vi "LowPassFilter.vi"(7 "Low-pass filter":T2={"Clip off ramp-up, 1/Fc"=1.0, "Double-pass in reverse"=TRUE, "IIR filter specifications"={"Topology"=enum."Butterworth", "Type"=enum."Lowpass", "Order"=1, "Lower Fc"=10000.0, "Upper Fc"=200.0, "PB Ripple"=1.0, "SB Attenuation"=60.0}} {"IIR filter specifications"."PB Ripple" format="%0.2f"; "IIR filter specifications"."Lower Fc" format="%0.2p"; "IIR filter specifications"."SB Attenuation" format="%0.2f"; "IIR filter specifications"."Upper Fc" format="%0.2p"}, 8 "error in (no error)":errorcluster, 9 "Settings":string, 11 "signal(s) in":waveform(dbl)[](array[waveform])) -> (0 "error out":errorcluster, 1 "Settings out":string, 3 "signal(s) out":waveform(dbl)[](array[waveform]), 4 "filter information":T1 {"phase H(w)"."df" format="%.2p"; "phase H(w)"."f0" format="%.2p"; "phase H(w)"."Phase H(w)" format="%.2p"; "magnitude H(w)"."df" format="%.2p"; "magnitude H(w)"."f0" format="%.2p"; "magnitude H(w)"."Mag H(w)" format="%.2p"})   [LabVIEW 2015]
uses:
  IIR Filter parameters.ctl
  <vilib>/measure/macond.llb/IIR Filter for N Chan.vi
  <vilib>/Waveform/WDTOps.llb/WDT Waveform Duration DBL.vi
  <vilib>/Waveform/WDTOps.llb/WDT Get Waveform Subset DBL.vi
  <vilib>/measure/NI_MAPro.lvlib
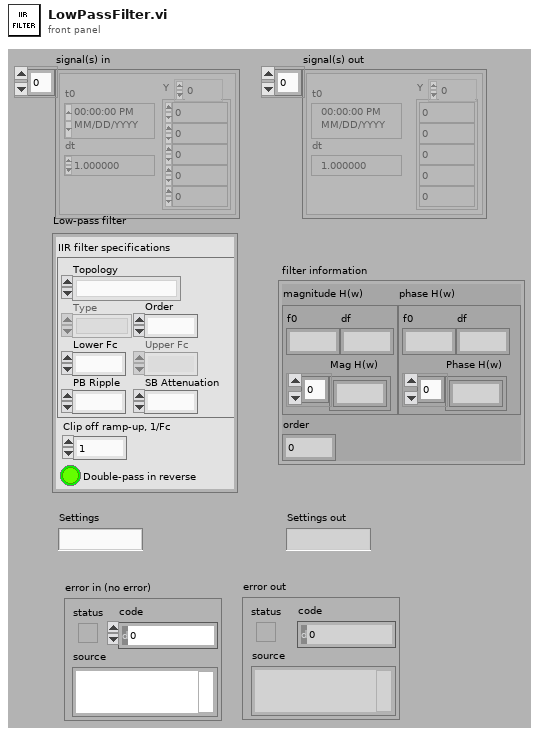
[diagram p1: front panel]
types:
  T1 = cluster{"magnitude H(w)":cluster{"f0":dbl, "df":dbl, "Mag H(w)":dbl[]}, "phase H(w)":cluster{"f0":dbl, "df":dbl, "Phase H(w)":dbl[]}, "order":i32}
  T2 = typedef "IIR Filter parameters.ctl" = cluster{"Clip off ramp-up, 1/Fc":dbl, "Double-pass in reverse":bool, "IIR filter specifications":cluster{"Topology":enum16{"Off", "Butterworth", "Chebyshev", "Inverse Chebyshev", "Elliptic", "Bessel"}, "Type":enum16{"Lowpass", "Highpass", "Bandpass", "Bandstop"}, "Order":i32, "Lower Fc":dbl, "Upper Fc":dbl, "PB Ripple":dbl, "SB Attenuation":dbl}}
  T3 = cluster{"Topology":enum16{"Off", "Butterworth", "Chebyshev", "Inverse Chebyshev", "Elliptic", "Bessel"}, "Type":enum16{"Lowpass", "Highpass", "Bandpass", "Bandstop"}, "Order":i32, "Lower Fc":dbl, "Upper Fc":dbl, "PB Ripple":dbl, "SB Attenuation":dbl}
  T4 = enum16{"Off", "Butterworth", "Chebyshev", "Inverse Chebyshev", "Elliptic", "Bessel"}
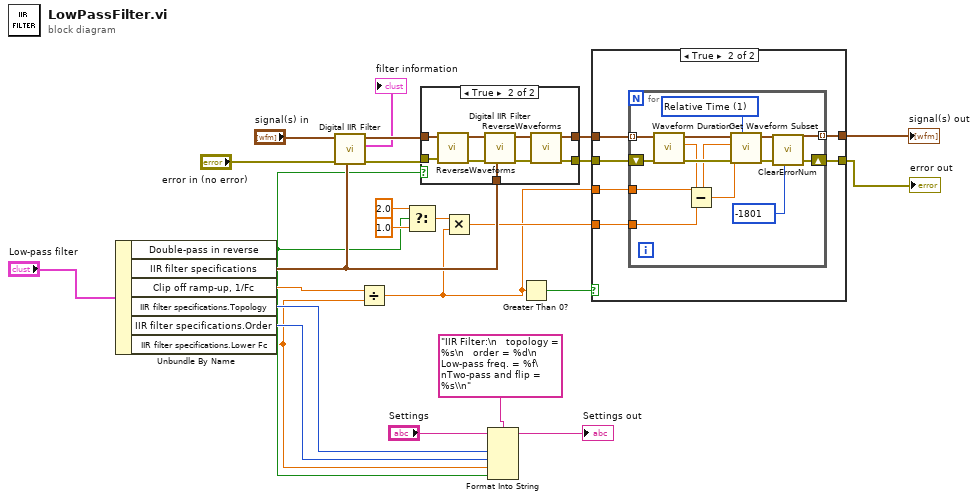
[diagram p0: block diagram]
diagram:
  n1 = Unbundle By Name("Low-pass filter") -> ("Double-pass in reverse"=w4:bool, "IIR filter specifications"=w21:T3, "Clip off ramp-up, 1/Fc"=w10:dbl, "IIR filter specifications.Topology"=w7:T4, "IIR filter specifications.Order"=w5:i32, "IIR filter specifications.Lower Fc"=w2:dbl)
  n2 = call-poly <vilib>:"Digital IIR Filter.vi"("IIR filter specifications"=w21, "error in (no error)"="error in (no error)", "signal(s) in"="signal(s) in") -> ("error out"=w24:errorcluster, "filter information"=→"filter information":T1, "signal(s) out"=w25:waveform(dbl)[])  [unwired: 3 in, 3 out]
  n3 = Divide(x=w10, y=w2) -> (x/y=w3:dbl)
  n4 = Select(t=2.0, s=w4, f=1.0) -> (s? t:f=w15:dbl)
  n5 = case shown="True" w4 {
    tunnel: w25 -> [w26 w34]
    tunnel: w24 -> [w27 w33]
    tunnel: [w27 w32] -> w19
    tunnel: [w26 w28] -> w20
    tunnel: w21 -> [_ w30]
    frame False {
    }
    frame True {
      n6 = call "ReverseWaveforms.vi"("signals in"=w34) -> ("signals out"=w29:waveform(dbl)[])  [unwired: 10 out]
      n7 = call-poly <vilib>:"Digital IIR Filter.vi"("IIR filter specifications"=w30, "error in (no error)"=w33, "signal(s) in"=w29) -> ("error out"=w32:errorcluster, "signal(s) out"=w31:waveform(dbl)[])  [unwired: 3 in, 4 out]
      n8 = call "ReverseWaveforms.vi"("signals in"=w31) -> ("signals out"=w28:waveform(dbl)[])  [unwired: 10 out]
    }
  }
  n9 = Multiply(x=w15, y=w3) -> (x*y=w14:dbl)
  n10 = Format Into String(format string="IIR Filter:\n   topology = %s\n   order = %d\n   Low-pass freq. = %f\nTwo-pass and flip = %s\\n", initial string="Settings", w7, w5, w2, w4) -> (resulting string=→"Settings out":string)  [unwired: 1 in, 1 out]
  n11 = Greater Than 0?(x=w3) -> (x > 0?=w13:bool)
  n12 = case shown="True" w13 {
    tunnel: w20 -> [w36 w42]
    tunnel: w19 -> [w35 w41]
    tunnel: [w36 w40] -> w18
    tunnel: w3 -> [_ w39]
    tunnel: w14 -> [_ w38]
    tunnel: [w35 w37] -> w11
    frame False {
    }
    frame True {
      n13 = for {
        tunnel: w42 -> [w50] mode=indexing
        shift-right: [w44] -> w37
        shift-left: w41 -> [w55]
        tunnel: [w53] -> w40 mode=indexing
        tunnel: w39 -> [w48]
        tunnel: w38 -> [w46]
        w51 = u16 1 items=["Samples", "Relative Time"] ("start/duration format")
        n14 = call-poly <vilib>:"Waveform Duration.vi"("error in (no error)"=w55, "waveform in"=w50) -> ("error out"=w52:errorcluster, "duration"=w47:dbl, "waveform out"=w49:waveform(dbl))  [unwired: 7 out]
        n15 = Subtract(x=w47, y=w46) -> (x-y=w45:dbl)
        n16 = call-poly <vilib>:"Get Waveform Subset.vi"("start/duration format"=w51, "error in (no error)"=w52, "duration"=w45, "start samples/time"=w48, "waveform in"=w49) -> ("error out"=w54:errorcluster, "waveform out"=w53:waveform(dbl))  [unwired: 3 out]
        n17 = call "ClearErrorNum.vi"("error in (no error)"=w54, "code"=-1801) -> ("error out"=w44:errorcluster)  [unwired: 7 in]
      }
    }
  }
  "signal(s) out" <- w18
  "error out" <- w11
